vi "Display Status.vi"(8 "error in (no error)":errorcluster, 10 "Status.Login Time":cluster{"minute":i32, "hour":i32}, 11 "Programing Logic in":refnum<class "Programing Logic.lvclass">) -> (0 "error out":errorcluster, 1 "commandValue":dbl, 2 "Status":T1, 3 "Programing Logic out":refnum<class "Programing Logic.lvclass">, 5 "Drives Connection":cluster{"Drive 1":bool, "Drive 2":bool})   [LabVIEW 2014, in "Programing Logic.lvclass"]
uses:
  Programing Logic.lvclass
  Programing Logic.lvclass/Programing Logic.ctl
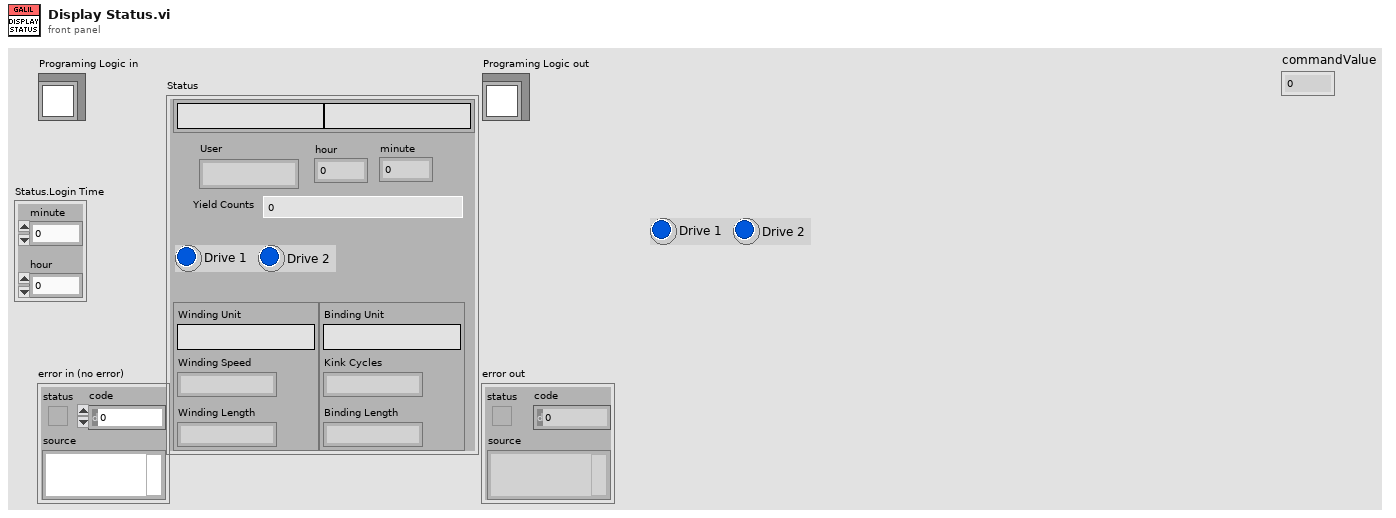
[diagram p1: front panel]
types:
  T1 = cluster{"Winding":cluster{"Winding Unit":string, "Winding Speed":string, "Winding Length":string}, "Binding":cluster{"Binding Unit":string, "Kink Cycles":string, "Binding Length":string}, "Yield Counts":dbl, "DataTime":cluster{"Date":string, "Time":string}, "User":string, "hour":i32, "minute":i32, "Drives Connection":cluster{"Drive 1":bool, "Drive 2":bool}}
  T2 = cluster{"Winding":cluster{"Winding Unit":string, "Winding Speed":string, "Winding Length":string}, "Binding":cluster{"Binding Unit":string, "Kink Cycles":string, "Binding Length":string}, "Yield Counts":dbl, "DataTime":cluster{"Date":string, "Time":string}, "User":string, "minute":i32, "hour":i32, "Drives Connection":cluster{"Drive 1":bool, "Drive 2":bool}}
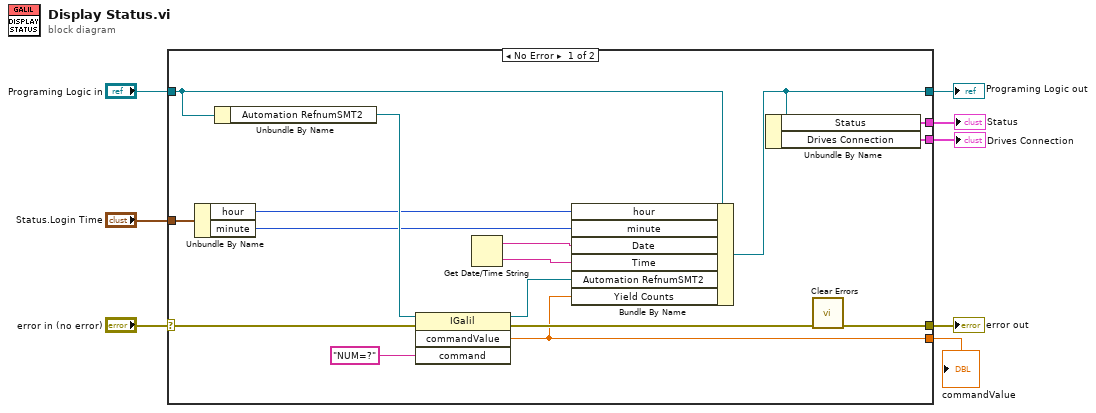
[diagram p0: block diagram]
diagram:
  n1 = case shown="No Error" "error in (no error)" {
    selector: "error in (no error)" -> [w24 w26]
    tunnel: [w16 w26] -> w7
    tunnel: [w19 w25] -> w5
    tunnel: "Programing Logic in" -> [w20 w25]
    tunnel: [w18 _] -> w4
    tunnel: "Status.Login Time" -> [w13 _]
    tunnel: [w10 _] -> w2
    tunnel: [w9 _] -> w1
    frame No Error {
      n2 = Unbundle By Name(w13) -> ("hour"=w12:i32, "minute"=w11:i32)
      n3 = Unbundle By Name(w20) -> ("Automation RefnumSMT2"=w22:refnum<k7>)
      n4 = invoke class="IGalil" method="commandValue"(reference=w22, error in=w24, "command"="NUM=?") -> (reference out=w21:refnum<k7>, error out=w17:errorcluster, "commandValue"=w10:dbl)  [unwired: 1 in, 1 out]
      n5 = Get Date/Time String() -> (date string=w15:string, time string=w14:string)  [unwired: 3 in]
      n6 = Bundle By Name(cluster=w20, "hour"=w12, "minute"=w11, "Date"=w15, "Time"=w14, "Automation RefnumSMT2"=w21, "Yield Counts"=w10) -> (w19:refnum<class "Programing Logic.lvclass">)
      n7 = Unbundle By Name(w19) -> ("Status"=w18:T2, "Drives Connection"=w9:cluster{"Drive 1":bool, "Drive 2":bool})
      n8 = call <vilib>:"Clear Errors.vi"("error in (no error)"=w17) -> ("error out"=w16:errorcluster)  [unwired: 5 in, 1 out]
    }
    frame Error {
    }
  }
  "error out" <- w7
  "Programing Logic out" <- w5
  "Status" <- w4
  "commandValue" <- w2
  "Drives Connection" <- w1
